vi "Untitled 1.vi"() -> ()   [LabVIEW 2011]
panel:
  out "dt":dbl format="%#_12g"
  in  "data":waveform(dbl)[](graph)
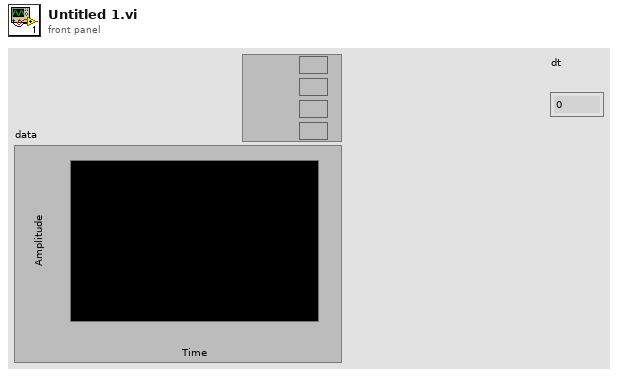
[diagram p1: front panel]
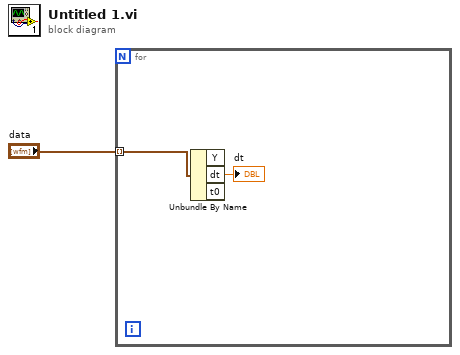
[diagram p0: block diagram]
diagram:
  n1 = for {
    tunnel: "data" -> [w3] mode=indexing
    n2 = Unbundle By Name(w3) -> ("dt"=→"dt":dbl)  [unwired: 2 out]
  }
